vi "gfitsio-read-column-i16-scalar.vi"(6 "row":i32, 7 "column":string, 8 "error in (no error)":errorcluster, 11 "gfits refnum":T1) -> (0 "error out":errorcluster, 2 "data":i16, 3 "dup gfits refnum":T1)   [LabVIEW 2011, in "gfitsio.lvlib"]
doc: "Read elements from an ASCII or binary table column."
uses:
  gfitsio.lvlib
  gfitsio-refnum.ctl
  cfitsio-hdutypes.ctl
  gfitsio.dll
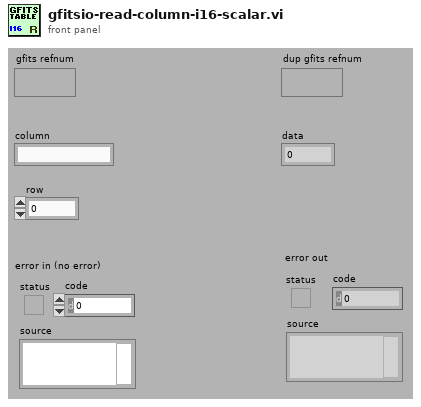
[diagram p1: front panel]
types:
  T1 = typedef "gfitsio.lvlib/gfitsio-refnum.ctl" = refnum<k1>
  T2 = typedef "gfitsio.lvlib/cfitsio-hdutypes.ctl" = i32
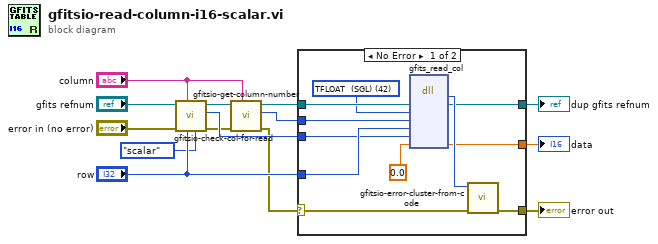
[diagram p0: block diagram]
diagram:
  n1 = call "gfitsio-check-col-for-read.vi"("expected dimensionality"=enum16{"scalar", "array"}."scalar", "row"="row", "column"="column", "error in (no error)"="error in (no error)", "gfits refnum"="gfits refnum") -> ("error out"=w5:errorcluster, "nelements"=w8:i32, "dup gfits refnum"=w7:T1)  [unwired: 4 in]
  n2 = call "gfitsio-get-column-number.vi"("column"="column", "error in (no error)"=w5, "gfits refnum"=w7) -> ("error out"=w4:errorcluster, "colnum"=w3:i32, "dup gfits refnum"=w6:T1)  [unwired: 6 in]
  n3 = case shown="No Error" w4 {
    selector: w4 -> [w25 w27]
    tunnel: [w24 w27] -> w14
    tunnel: w6 -> [w21 w26]
    tunnel: [w22 w26] -> w13
    tunnel: "row" -> [w17 _]
    tunnel: w3 -> [w18 _]
    tunnel: [w19 _] -> w12
    tunnel: w8 -> [w15 _]
    frame No Error {
      w16 = T2 42 items=["TBIT"=1, "TBYTE  (U8)"=11, "TSBYTE  (I8)"=12, "TLOGICAL"=14, "TSTRING"=16, "TUSHORT  (U16)"=20, "TSHORT  (I16)"=21, "TUINT"=31, "TULONG  (U32)"=40, "TLONG  (I32)"=41, "TFLOAT  (SGL)"=42, "TLONGLONG  (I64)"=81, "TDOUBLE"=82, "TCOMPLEX  (CSG)"=83, "TDOUBLECOMPLEX  (CDB)"=163] ("cfitsio datatype")
      n4 = dll-call lib="C:/BonOMM/BonOMM-SAOMM/SubVIs/gfitsio/gfitsio.dll" fn="gfits_read_col"("dup gfits refnum"=w21, "datatype"=w16, "colnum"=w18, "row"=w17, "nelements"=w15, "data"=sgl 0.0) -> (w23:i32, "dup gfits refnum"=w22:T1, "data"=w19:sgl)  [unwired: 7 in, 2 out]
      n5 = call "gfitsio-error-cluster-from-code.vi"("error in (no error)"=w25, "error code"=w23) -> ("error out"=w24:errorcluster)  [unwired: 9 in]
    }
    frame Error {
    }
  }
  "error out" <- w14
  "dup gfits refnum" <- w13
  "data" <- w12
